vi "WriteIOValues b2g2.vi"(2 "error in":errorcluster, 3 "Output - Cluster b2g2":T1 {"TS-5 [°C]" format="%#.2g"; "pHS-1 [pH]" format="%.2g"; "TS-4 [°C]" format="%#.2g"; "FS-2 [l]" format="%.2g"; "FS-1 [l]" format="%.2g"; "DS-1 [bar]" format="%#.2g"; "DFS-1 [l/min]" format="%#.2g"; "FS-3 [l]" format="%.2g"; "DFS-1 [dl]" format="%.0g"}, 4 "input cluster":T2 {"Zirkulationgeschw. [l/min]" format="%.2g"; "FS-1 [l]" format="%_3g"; "Hysterese [°C]" format="%.2g"; "Dosiergeschw. [l/min]" format="%.2g"; "Dosiermenge [l]" format="%.2g"; "Druck I" format="%_3g"; "Füllstand  P" max=100 step=1 format="%#_3g"; "P-4 Drehzahl [%]" max=100 step=1 format="%#_3g"; "V-15 [%]" max=100 step=1 format="%_1g"; "V-13 [%]" max=100 step=1 format="%_1g"}) -> (0 "error out":errorcluster, 1 "output cluster":T1 {"TS-5 [°C]" format="%#.2g"; "pHS-1 [pH]" format="%.2g"; "TS-4 [°C]" format="%#.2g"; "FS-2 [l]" format="%.2g"; "FS-1 [l]" format="%.2g"; "DS-1 [bar]" format="%#.2g"; "DFS-1 [l/min]" format="%#.2g"; "FS-3 [l]" format="%.2g"; "DFS-1 [dl]" format="%.0g"})   [LabVIEW 2011]
uses:
  Input - Cluster b2g2.ctl
  Output - Cluster b2g2.ctl
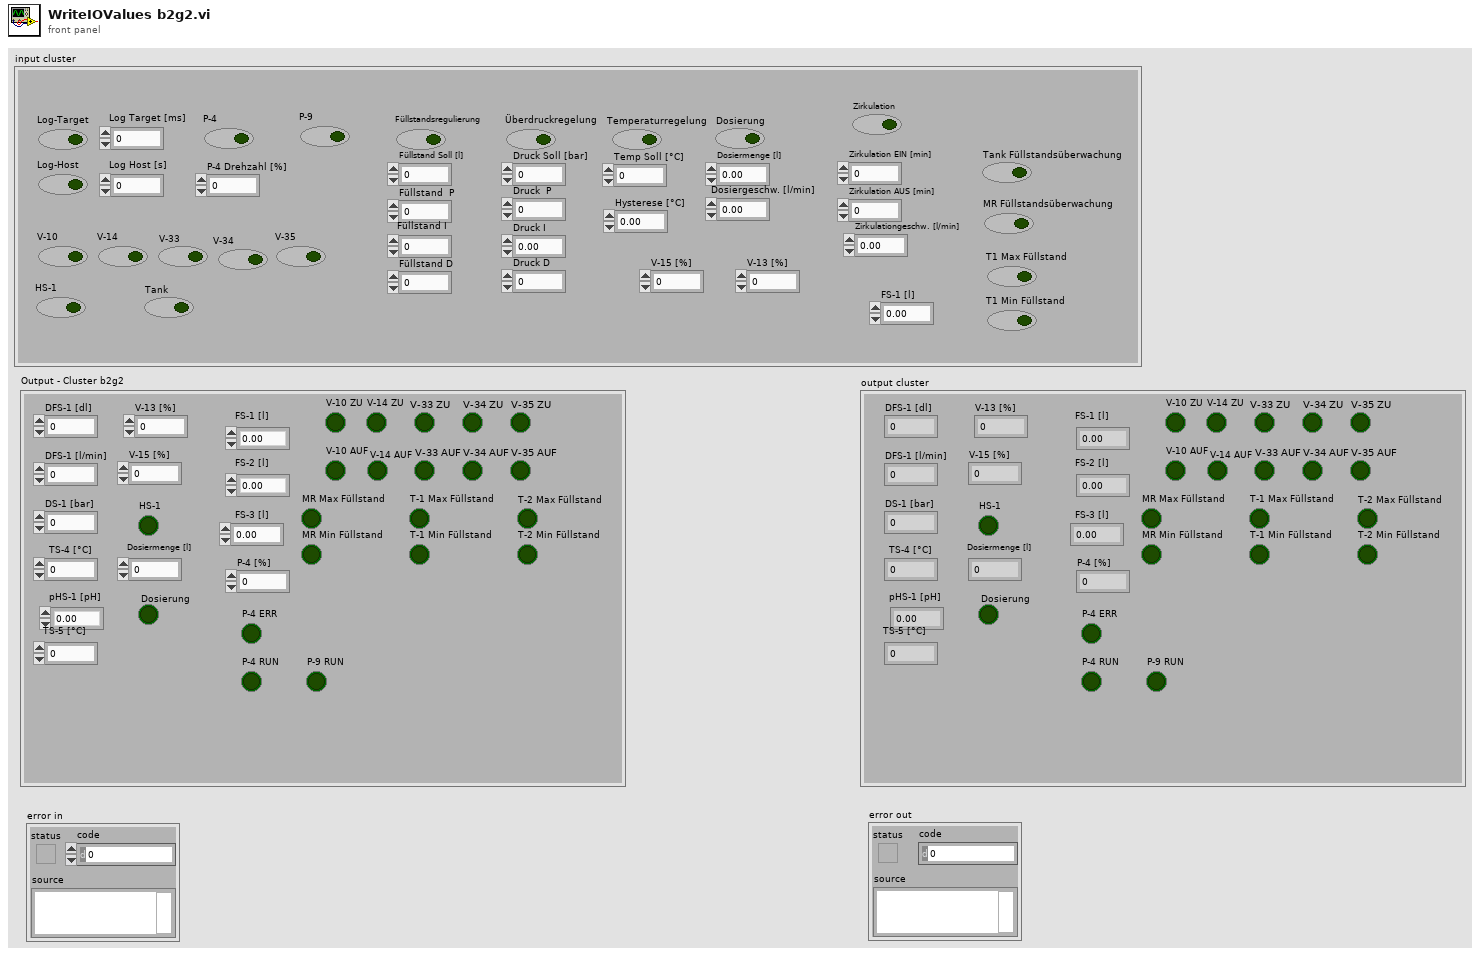
[diagram p1: front panel]
types:
  T1 = typedef "Output - Cluster b2g2.ctl" = cluster{"DFS-1 [dl]":u64, "FS-3 [l]":dbl, "DFS-1 [l/min]":dbl, "DS-1 [bar]":dbl, "V-10 ZU":bool, "V-14 ZU":bool, "FS-1 [l]":dbl, "FS-2 [l]":dbl, "TS-4 [°C]":dbl, "HS-1":bool, "V-13 [%]":u8, "V-15 [%]":u8, "P-4 [%]":u8, "Dosierung":bool, "MR Max Füllstand":bool, "MR Min Füllstand":bool, "Dosiermenge [l]":sgl, "V-14 AUF":bool, "V-10 AUF":bool, "T-1 Max Füllstand":bool, "T-1 Min Füllstand":bool, "T-2 Max Füllstand":bool, "T-2 Min Füllstand":bool, "pHS-1 [pH]":dbl, "P-4 RUN":bool, "V-33 AUF":bool, "V-33 ZU":bool, "V-34 AUF":bool, "V-34 ZU":bool, "P-4 ERR":bool, "TS-5 [°C]":dbl, "V-35 AUF":bool, "V-35 ZU":bool, "P-9 RUN":bool}
  T2 = typedef "Input - Cluster b2g2.ctl" = cluster{"V-13 [%]":u8, "V-15 [%]":u8, "Log-Target":bool, "P-4":bool, "P-4 Drehzahl [%]":u8, "Temperaturregelung":bool, "Überdruckregelung":bool, "Füllstandsregulierung":bool, "V-10":bool, "Log-Host":bool, "V-14":bool, "HS-1":bool, "Füllstand  P":sgl, "Füllstand I":sgl, "Füllstand D":sgl, "Füllstand Soll [l]":sgl, "Druck  P":sgl, "Druck I":sgl, "Druck D":sgl, "Druck Soll [bar]":sgl, "Temp Soll [°C]":sgl, "Dosierung":bool, "Dosiermenge [l]":sgl, "Dosiergeschw. [l/min]":sgl, "Tank":bool, "Hysterese [°C]":sgl, "MR Füllstandsüberwachung":bool, "Tank Füllstandsüberwachung":bool, "Log Target [ms]":u32, "Log Host [s]":u32, "Zirkulation EIN [min]":u8, "Zirkulation AUS [min]":u8, "Zirkulation":bool, "V-33":bool, "V-34":bool, "V-35":bool, "T1 Max Füllstand":bool, "T1 Min Füllstand":bool, "FS-1 [l]":sgl, "P-9":bool, "Zirkulationgeschw. [l/min]":sgl}
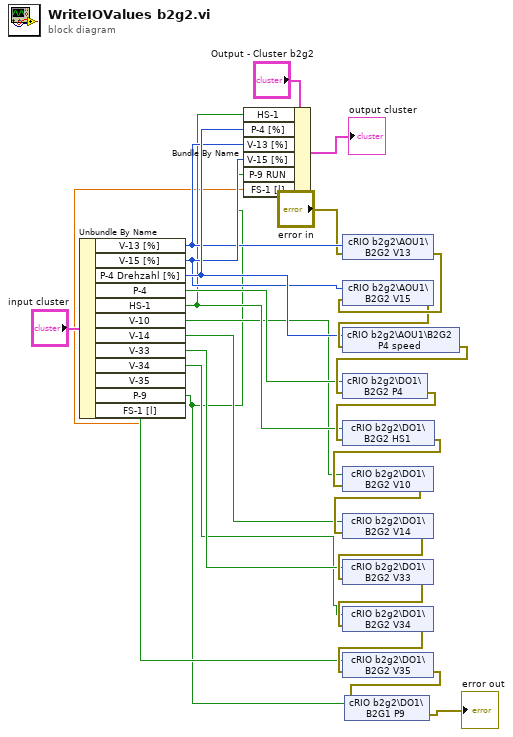
[diagram p0: block diagram]
diagram:
  n1 = Unbundle By Name("input cluster") -> ("V-13 [%]"=w16:u8, "V-15 [%]"=w17:u8, "P-4 Drehzahl [%]"=w21:u8, "P-4"=w19:bool, "HS-1"=w11:bool, "V-10"=w9:bool, "V-14"=w8:bool, "V-33"=w7:bool, "V-34"=w6:bool, "V-35"=w5:bool, "P-9"=w2:bool, "FS-1 [l]"=w1:sgl)
  n2 = Bundle By Name(cluster="Output - Cluster b2g2", "HS-1"=w11, "P-4 [%]"=w21, "V-13 [%]"=w16, "V-15 [%]"=w17, "P-9 RUN"=w2, "FS-1 [l]"=w1) -> (→"output cluster":T1)
  n3 = shared-variable "cRIO b2g2\\AOU1\\B2G2 V13"(w16, error in="error in") -> (error out=w27:errorcluster)
  n4 = shared-variable "cRIO b2g2\\AOU1\\B2G2 V15"(w17, error in=w27) -> (error out=w26:errorcluster)
  n5 = shared-variable "cRIO b2g2\\AOU1\\B2G2 P4 speed"(w21, error in=w26) -> (error out=w25:errorcluster)
  n6 = shared-variable "cRIO b2g2\\DO1\\B2G2 P4"(w19, error in=w25) -> (error out=w20:errorcluster)
  n7 = shared-variable "cRIO b2g2\\DO1\\B2G2 HS1"(w11, error in=w20) -> (error out=w10:errorcluster)
  n8 = shared-variable "cRIO b2g2\\DO1\\B2G2 V10"(w9, error in=w10) -> (error out=w23:errorcluster)
  n9 = shared-variable "cRIO b2g2\\DO1\\B2G2 V14"(w8, error in=w23) -> (error out=w22:errorcluster)
  n10 = shared-variable "cRIO b2g2\\DO1\\B2G2 V33"(w7, error in=w22) -> (error out=w18:errorcluster)
  n11 = shared-variable "cRIO b2g2\\DO1\\B2G2 V34"(w6, error in=w18) -> (error out=w15:errorcluster)
  n12 = shared-variable "cRIO b2g2\\DO1\\B2G2 V35"(w5, error in=w15) -> (error out=w4:errorcluster)
  n13 = shared-variable "cRIO b2g2\\DO1\\B2G1 P9"(w2, error in=w4) -> (error out=→"error out":errorcluster)
